vi "FTW-Example-SLASD-Core-Process.vi"() -> ()   [LabVIEW 2013, in "FTW-Example-SLASD-Core.lvclass"]
uses:
  FTW-Example-SLASD-Core.lvclass
  FTW-Example-SLASD-Core.lvclass/FTW-Example-SLASD-Core.ctl
  Actor/src/Instance/FTW-ActorInstance.lvclass/FTW-ActorInstance.ctl
  <vilib>/nisyscfg/Close (Hardware).vi
  <vilib>/nisyscfg/Close (System).vi
  <vilib>/nisyscfg/Find Hardware.vi
  Actor/src/JobSequencer/FTW-SEQ-Current.vi
  Actor/src/Instance/FTW-ActorInstance.lvclass
  Actor/src/Message/Request/FTW-Message-IncomingRequest.lvclass
  Actor/src/Ether/FTW-Ether.lvclass
  <vilib>/nisyscfg/nisyscfg.lvlib
  <resource>/objmgr/nisysapi.rc
panel:
  out "error out":errorcluster
  out "System Status":T1
  out "Elapsed Time":dbl format="%.6f sec"
  in  "Stop Button":bool
  # "avoid using Abort unless absolutely necessary"
  # "use this button to stop\nthe actor in RT dev mode\nsince user input events\ndo not work on RT"
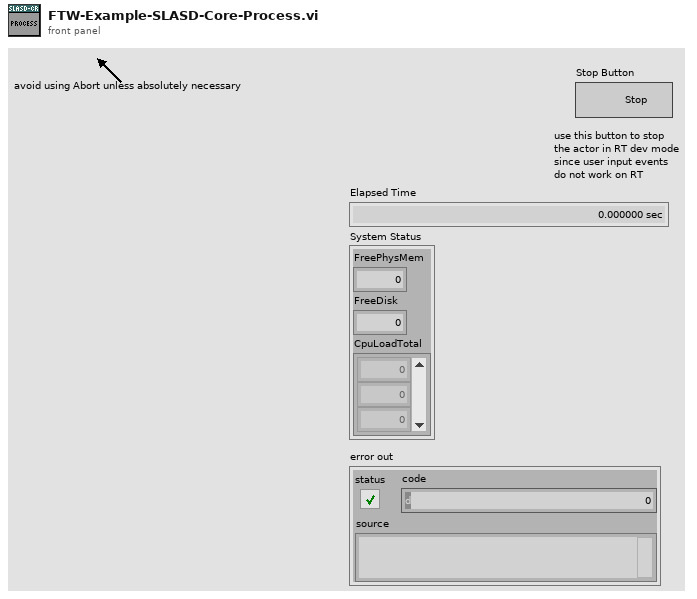
[diagram p1: front panel]
types:
  T1 = cluster{"FreePhysMem":dbl, "FreeDisk":dbl, "CpuLoadTotal":u32[]}
  T2 = cluster{"Incoming Requests":refnum<event-registration>, "Additional Registration Types":refnum<event-registration>}
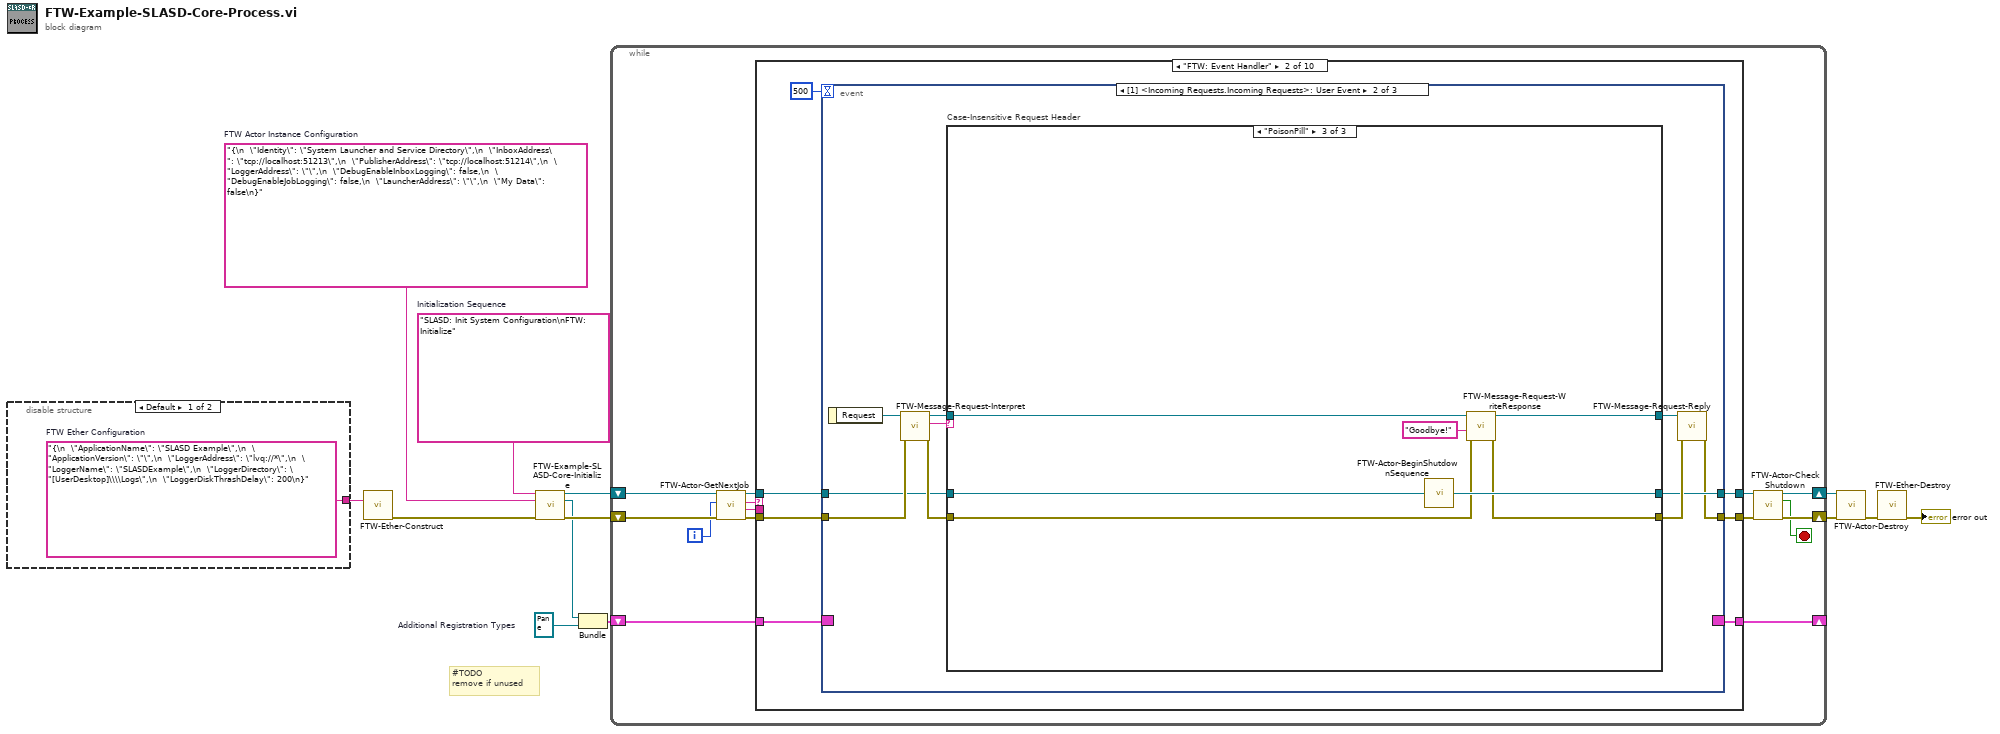
[diagram p0: block diagram]
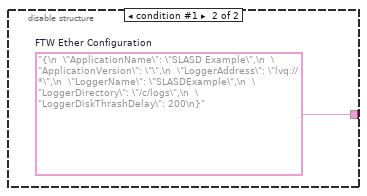
[diagram p2: hidden frame]
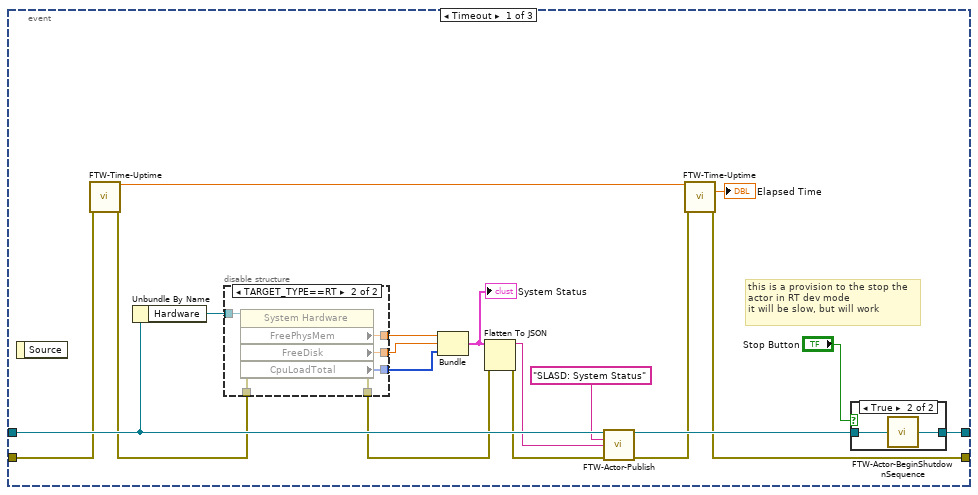
[diagram p4: hidden frame]
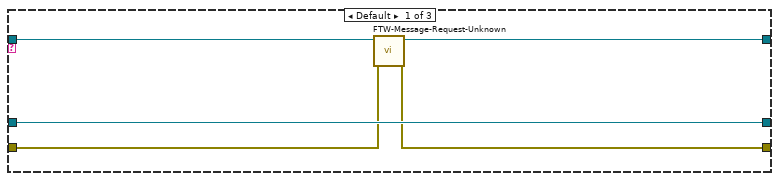
[diagram p7: hidden frame]
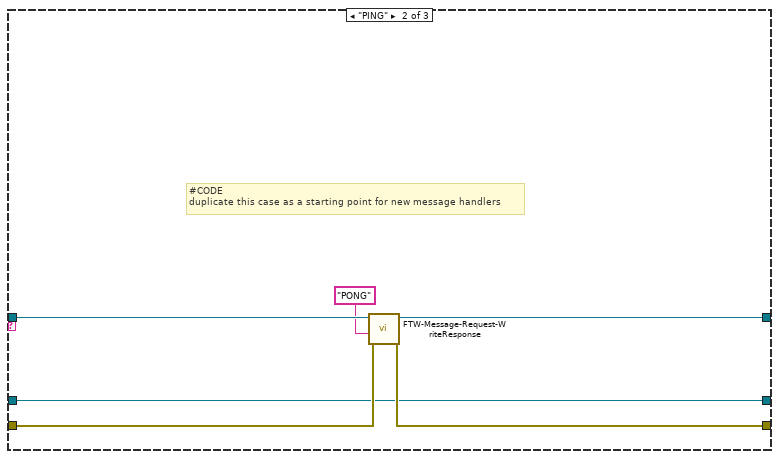
[diagram p8: hidden frame]
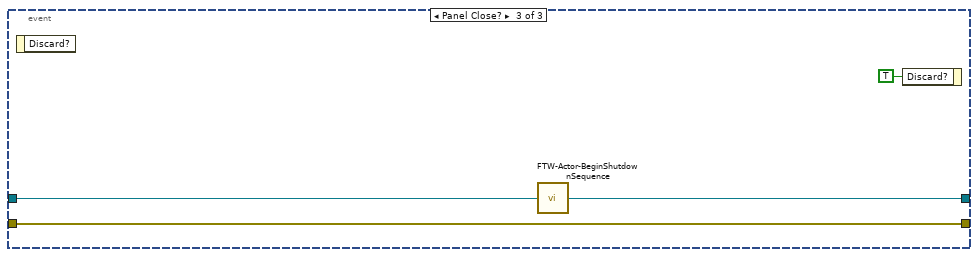
[diagram p9: hidden frame]
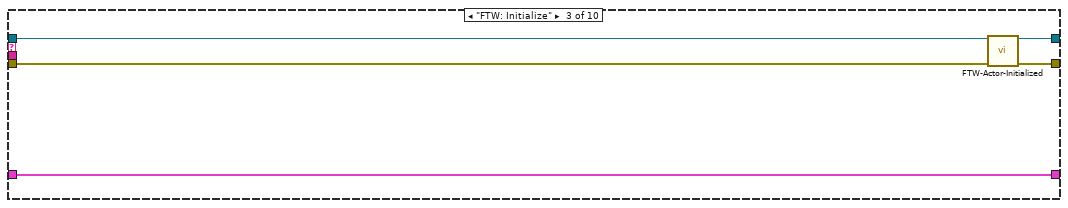
[diagram p10: hidden frame]
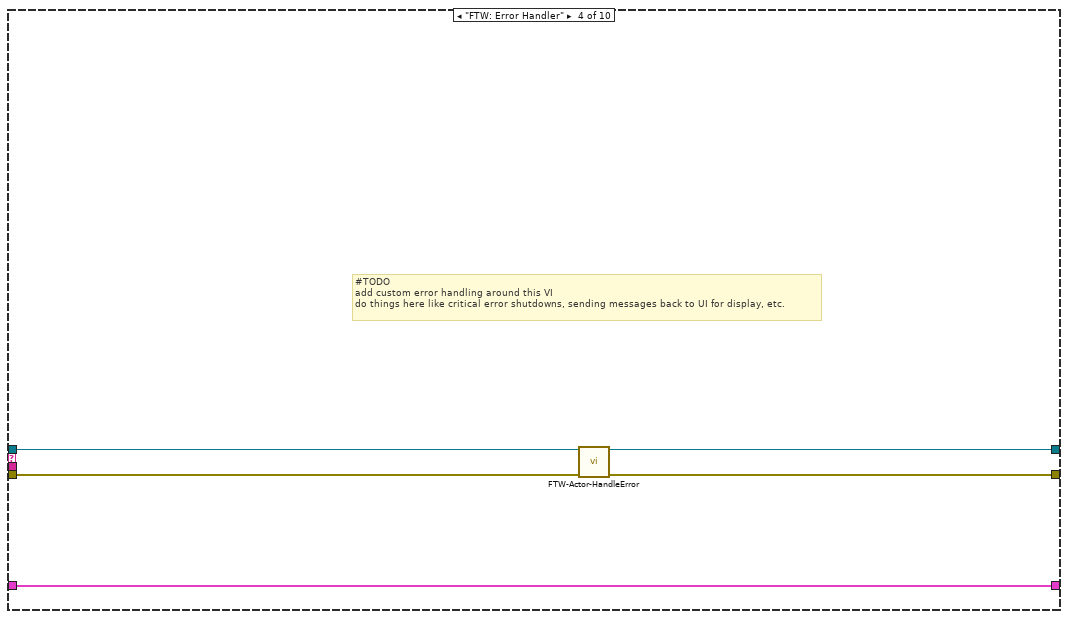
[diagram p11: hidden frame]
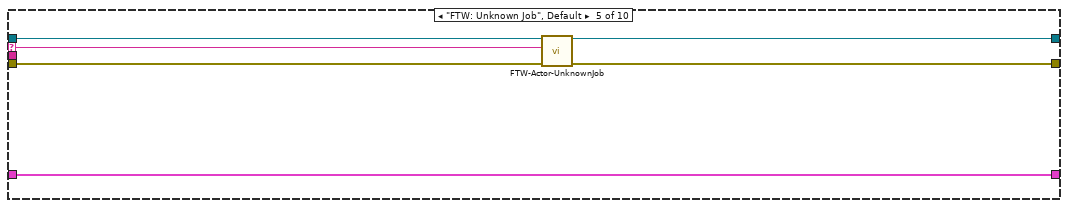
[diagram p12: hidden frame]
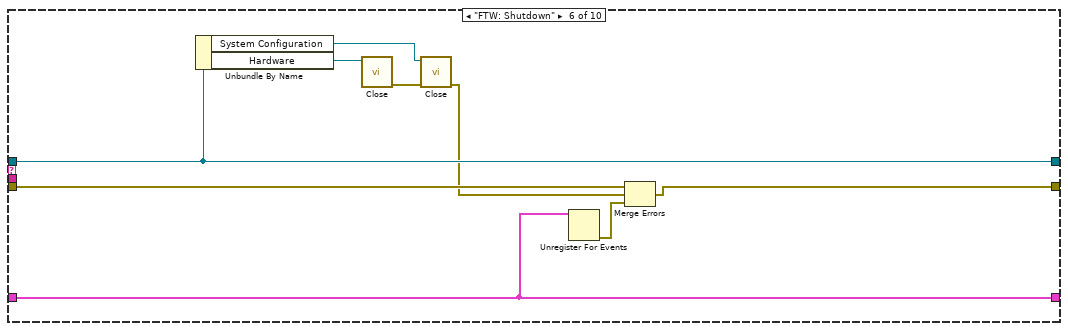
[diagram p13: hidden frame]
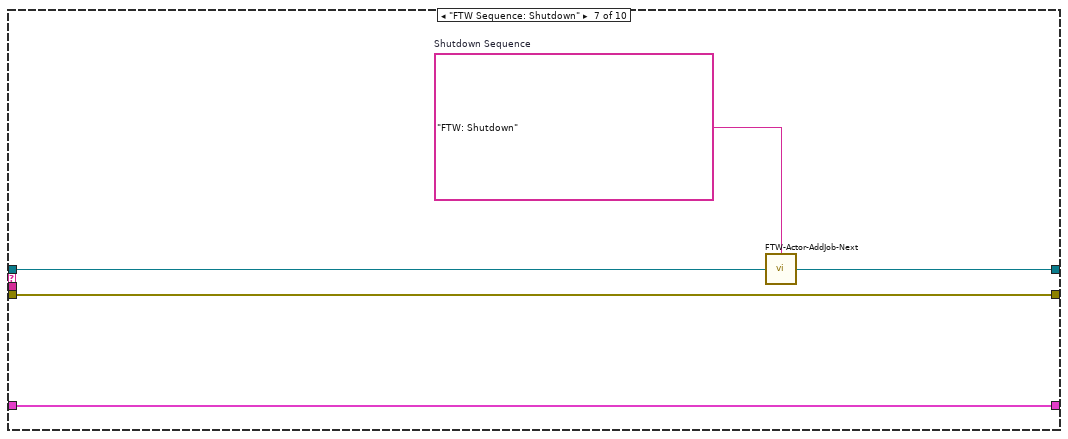
[diagram p14: hidden frame]
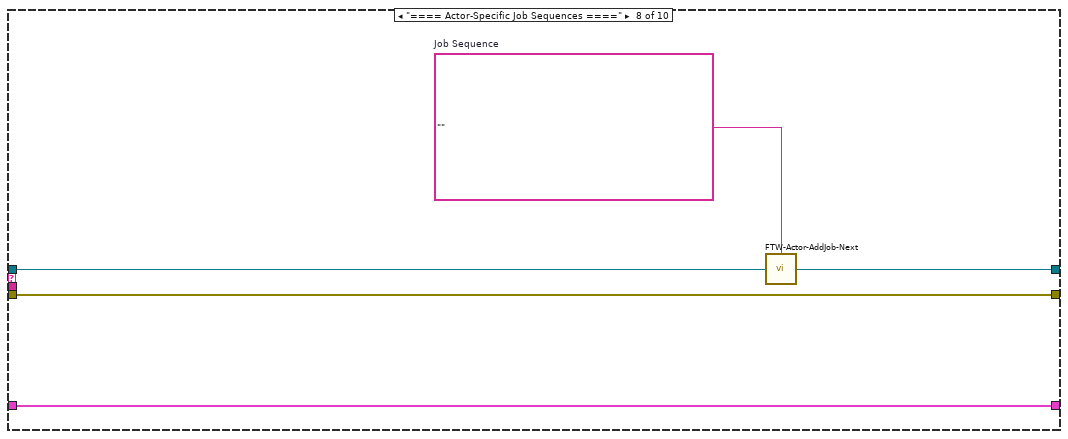
[diagram p15: hidden frame]
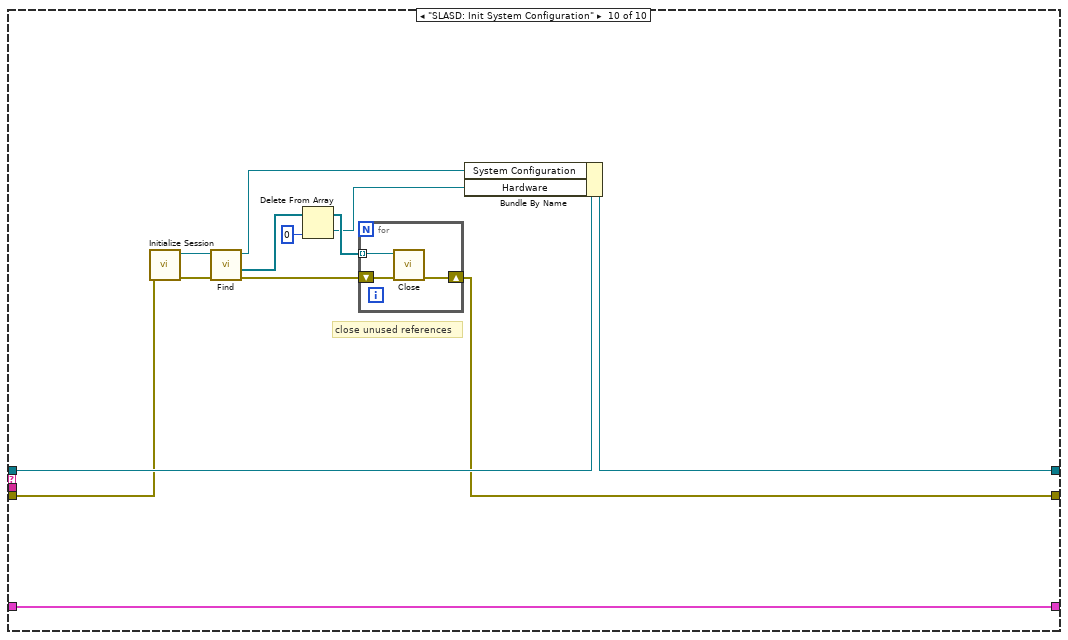
[diagram p17: hidden frame]
diagram:
  w5 = "{\n  \"Identity\": \"System Launcher and Service Directory\",\n  \"InboxAddress\": \"tcp://localhost:51213\",\n  \"PublisherAddress\": \"tcp://localhost:51214\",\n  \"LoggerAddress\": \"\",\n  \"DebugEnableInboxLogging\": false,\n  \"DebugEnableJobLogging\": false,\n  \"LauncherAddress\": \"\",\n  \"My Data\": false\n}"  # FTW Actor Instance Configuration
  w7 = refnum<event-registration> refnum  # Additional Registration Types
  w8 = "SLASD: Init System Configuration\nFTW: Initialize"  # Initialization Sequence
  # "#TODO\nremove if unused"
  n1 = disable-structure shown="Default" {
    disable-tunnel: [w14 w15] -> w2
    frame condition #0 (active) {
      w14 = "{\n  \"ApplicationName\": \"SLASD Example\",\n  \"ApplicationVersion\": \"\",\n  \"LoggerAddress\": \"lvq://*\",\n  \"LoggerName\": \"SLASDExample\",\n  \"LoggerDirectory\": \"[UserDesktop]\\\\Logs\",\n  \"LoggerDiskThrashDelay\": 200\n}"  # FTW Ether Configuration
    }
    frame condition #1 {
      w15 = "{\n  \"ApplicationName\": \"SLASD Example\",\n  \"ApplicationVersion\": \"\",\n  \"LoggerAddress\": \"lvq://*\",\n  \"LoggerName\": \"SLASDExample\",\n  \"LoggerDirectory\": \"/c/logs\",\n  \"LoggerDiskThrashDelay\": 200\n}"  # FTW Ether Configuration
    }
  }
  n2 = call "FTW-Ether-Construct.vi"("FTW Ether Configuration"=w2) -> ("error out"=w3:errorcluster)  [unwired: 14 in]
  n3 = call "FTW-Example-SLASD-Core-Initialize.vi"("Initialization Sequence"=w8, "FTW Actor Instance Configuration"=w5, "error in (no error)"=w3) -> ("Actor Template-Core out"=w13:refnum<class "FTW-Example-SLASD-Core.lvclass">, "Incoming Requests"=w4:refnum<event-registration>, "error out"=w9:errorcluster)  [unwired: 10 in]
  n4 = Bundle("Incoming Requests"=w4, "Additional Registration Types"=w7) -> (w6:T2)  [unwired: 1 in]
  n5 = while {
    shift-right: [w19] -> w11
    shift-left: w9 -> [w26]
    shift-right: [w16] -> _
    shift-left: w6 -> [w29]
    shift-right: [w21] -> w12
    shift-left: w13 -> [w28]
    i -> [w17]
    stop <- w18 stop-if-true
    n6 = call "FTW-Actor-GetNextJob.vi"("error in"=w26, "Jobs Performed"=w17, "FTW Actor Instance"=w28) -> ("error out"=w25:errorcluster, "Job Data"=w23:string, "Job Name"=w24:string, "FTW Actor Instance out"=w27:refnum<class "FTW-Example-SLASD-Core.lvclass">)  [unwired: 5 in]
    n7 = case shown="\"FTW: Event Handler\"" w24 {
      selector: w24 -> [_ _ _ _ w111 _ _ _ _ _]
      tunnel: [w31 w39 w101 w106 w114 w124 w129 w134 w138 w142] -> w20
      tunnel: w25 -> [w31 w38 w104 w108 w115 w125 w129 w134 w138 w143]
      tunnel: w29 -> [w32 w34 w105 w110 w116 w122 w130 w135 w137 w151]
      tunnel: [w32 w37 w105 w110 w116 w122 w130 w135 w137 w151] -> w16
      tunnel: w23 -> [_ _ _ _ _ _ _ _ _ _]
      tunnel: [w30 w36 w102 w107 w112 w121 w127 w132 w136 w141] -> w22
      tunnel: w27 -> [w30 w35 w103 w109 w113 w121 w128 w133 w136 w150]
      frame "==== Featherweight Framework Jobs ====" {
      }
      frame "FTW: Event Handler" {
        n8 = event shown="[1] <Incoming Requests.Incoming Requests>: User Event" {
          selector: w34 -> [_ _ _]
          dyn-events: [_ _ _] -> w37
          timeout: 500 -> [_ _ _]
          tunnel: [w42 w71 w99] -> w39
          tunnel: w38 -> [w56 w70 w99]
          tunnel: [w45 w72 w97] -> w36
          tunnel: w35 -> [w58 w69 w98]
          event Timeout {
            # "this is a provision to the stop the\nactor in RT dev mode\nit will be slow, but will work"
            n9 = event-data() -> ()  [unwired: 1 in, 1 out]
            n10 = call "FTW-Time-Uptime.vi"("error in"=w56) -> ("Current Uptime"=w41:dbl, "error out"=w43:errorcluster)  [unwired: 12 in, 1 out]
            n11 = Unbundle By Name(w58) -> ("Hardware"=w57:refnum<k20>)
            n12 = disable-structure shown="TARGET_TYPE==RT" {
              disable-tunnel: w43 -> [w62 w68]
              disable-tunnel: [_ w67] -> w50
              disable-tunnel: w57 -> [_ w66]
              disable-tunnel: [_ w65] -> w51
              disable-tunnel: [_ w64] -> w52
              disable-tunnel: [w62 w63] -> w49
              frame condition #0 (active) {
              }
              frame condition #1 {
                n13 = property class="System Hardware"(reference=w66, error in=w68) -> (error out=w63:errorcluster, "FreePhysMem"=w64:dbl, "FreeDisk"=w65:dbl, "CpuLoadTotal"=w67:u32[])  [unwired: 1 out]
              }
            }
            n14 = Bundle("FreePhysMem"=w52, "FreeDisk"=w51, "CpuLoadTotal"=w50) -> (w47:T1)  [unwired: 1 in]
            "System Status" <- w47
            n15 = Flatten To JSON(anything=w47, error in (no error)=w49) -> (JSON string=w46:string, 11:w48:errorcluster)  [unwired: 1 in]
            n16 = call "FTW-Actor-Publish.vi"("FTW-ActorInstance In"=w58, "Message Header"="SLASD: System Status", "Message Body"=w46, "error in (no error)"=w48) -> ("FTW-ActorInstance Out"=w55:refnum<class "FTW-Example-SLASD-Core.lvclass">, "error out"=w54:errorcluster)  [unwired: 10 in]
            n17 = call "FTW-Time-Uptime.vi"("Previous Uptime"=w41, "error in"=w54) -> ("Elapsed Time"=→"Elapsed Time":dbl, "error out"=w42:errorcluster)  [unwired: 11 in, 1 out]
            n18 = case shown="True" "Stop Button" {
              tunnel: w55 -> [w59 w61]
              tunnel: [w59 w60] -> w45
              frame False {
              }
              frame True {
                n19 = call "FTW-Actor-BeginShutdownSequence.vi"("FTW Actor Instance"=w61) -> ("FTW Actor Instance out"=w60:refnum<class "FTW-Example-SLASD-Core.lvclass">)  [unwired: 3 in]
              }
            }
          }
          event User Event {
            n20 = event-data() -> ("Request"=w73:refnum<class "FTW-Message-IncomingRequest.lvclass">)  [unwired: 1 in]
            n21 = call "FTW-Message-Request-Interpret.vi"("error in"=w70, "FTW Incoming Request"=w73) -> ("error out"=w78:errorcluster, "Request Header"=w76:string, "FTW Incoming Request out"=w75:refnum<class "FTW-Message-IncomingRequest.lvclass">)  [unwired: 7 in]
            n22 = case "Case-Insensitive Request Header" shown="\"PoisonPill\"" w76 {
              tunnel: [w81 w87 w93] -> w77
              tunnel: w78 -> [w82 w88 w95]
              tunnel: [w83 w86 w96] -> w72
              tunnel: w69 -> [w83 w86 w94]
              tunnel: w75 -> [w80 w89 w92]
              tunnel: [w79 w85 w91] -> w74
              frame Default {
                n23 = call "FTW-Message-Request-Unknown.vi"("error in"=w82, "FTW Incoming Request"=w80) -> ("error out"=w81:errorcluster, "FTW Incoming Request Out"=w79:refnum<class "FTW-Message-IncomingRequest.lvclass">)  [unwired: 8 in]
              }
              frame "PING" {
                # "#CODE\nduplicate this case as a starting point for new message handlers"
                n24 = call "FTW-Message-Request-WriteResponse.vi"("error in"=w88, "Response Body"="PONG" ("Response Header"), "FTW Incoming Request"=w89) -> ("error out"=w87:errorcluster, "FTW Incoming Request out"=w85:refnum<class "FTW-Message-IncomingRequest.lvclass">)  [unwired: 7 in]
              }
              frame "PoisonPill" {
                n25 = call "FTW-Actor-BeginShutdownSequence.vi"("FTW Actor Instance"=w94) -> ("FTW Actor Instance out"=w96:refnum<class "FTW-Example-SLASD-Core.lvclass">)  [unwired: 3 in]
                n26 = call "FTW-Message-Request-WriteResponse.vi"("error in"=w95, "Response Body"="Goodbye!", "FTW Incoming Request"=w92) -> ("error out"=w93:errorcluster, "FTW Incoming Request out"=w91:refnum<class "FTW-Message-IncomingRequest.lvclass">)  [unwired: 7 in]
              }
            }
            n27 = call "FTW-Message-Request-Reply.vi"("error in"=w77, "FTW Incoming Request"=w74) -> ("error out"=w71:errorcluster)  [unwired: 8 in, 1 out]
          }
          event Panel Close? {
            n28 = event-data() -> ()  [unwired: 1 in, 1 out]
            n29 = call "FTW-Actor-BeginShutdownSequence.vi"("FTW Actor Instance"=w98) -> ("FTW Actor Instance out"=w97:refnum<class "FTW-Example-SLASD-Core.lvclass">)  [unwired: 3 in]
            n30 = event-data("Discard?"=TRUE) -> ()  [unwired: 1 in, 1 out]
          }
        }
      }
      frame "FTW: Initialize" {
        n31 = call-dynamic "FTW-Actor-Initialized.vi"("FTW Actor Instance"=w103, "error in"=w104) -> ("FTW Actor Instance out"=w102:refnum<class "FTW-Example-SLASD-Core.lvclass">, "error out"=w101:errorcluster)  [unwired: 12 in]
      }
      frame "FTW: Error Handler" {
        # "#TODO\nadd custom error handling around this VI\ndo things here like critical error shutdowns, sending messages back to UI for display, etc."
        n32 = call-dynamic "FTW-Actor-HandleError.vi"("FTW Actor Instance"=w109, "error in"=w108) -> ("FTW Actor Instance out"=w107:refnum<class "FTW-Example-SLASD-Core.lvclass">, "error out"=w106:errorcluster)  [unwired: 11 in, 1 out]
      }
      frame "FTW: Unknown Job", Default {
        n33 = call-dynamic "FTW-Actor-UnknownJob.vi"("FTW Actor Instance"=w113, "Unknown Job"=w111, "error in"=w115) -> ("FTW Actor Instance out"=w112:refnum<class "FTW-Example-SLASD-Core.lvclass">, "error out"=w114:errorcluster)  [unwired: 11 in]
      }
      frame "FTW: Shutdown" {
        n34 = Unbundle By Name(w121) -> ("System Configuration"=w118:refnum<k21>, "Hardware"=w120:refnum<k20>)
        n35 = call-poly <vilib>:"Close.vi"("resource in"=w120) -> ("error out"=w119:errorcluster)  [unwired: 10 in]
        n36 = call-poly <vilib>:"Close.vi"("error in (no error)"=w119, "session in"=w118) -> ("error out"=w117:errorcluster)  [unwired: 9 in]
        n37 = Unregister For Events(event registration refnum=w122) -> (error out=w123:errorcluster)  [unwired: 1 in]
        n38 = Merge Errors(w125, w117, w123) -> (w124:errorcluster)
      }
      frame "FTW Sequence: Shutdown" {
        w126 = "FTW: Shutdown"  # Shutdown Sequence
        n39 = call "FTW-Actor-AddJob-Next.vi"("Add Next in Job Queue"=w126, "FTW Actor Instance"=w128) -> ("FTW Actor Instance out"=w127:refnum<class "FTW-Example-SLASD-Core.lvclass">)  [unwired: 2 in]
      }
      frame "==== Actor-Specific Job Sequences ====" {
        w131 = ""  # Job Sequence
        n40 = call "FTW-Actor-AddJob-Next.vi"("Add Next in Job Queue"=w131, "FTW Actor Instance"=w133) -> ("FTW Actor Instance out"=w132:refnum<class "FTW-Example-SLASD-Core.lvclass">)  [unwired: 2 in]
      }
      frame "==== Actor-Specific Jobs ====" {
      }
      frame "SLASD: Init System Configuration" {
        # "close unused references"
        n41 = call <vilib>:"Initialize Session.vi"("error in (no error)"=w143) -> ("error out"=w149:errorcluster, "session out"=w148:refnum<k21>)  [unwired: 9 in]
        n42 = call-poly <vilib>:"Find.vi"("error in (no error)"=w149, "session in"=w148) -> ("error out"=w145:errorcluster, "resources out"=w147:refnum<k20>[], "session out"=w140:refnum<k21>)  [unwired: 6 in, 1 out]
        n43 = Delete From Array(array=w147, index=0) -> (deleted portion=w139:refnum<k20>, array with subset deleted=w144:refnum<k20>[])  [unwired: 1 in]
        n44 = for {
          tunnel: w144 -> [w154] mode=indexing
          shift-right: [w152] -> w142
          shift-left: w145 -> [w153]
          n45 = call-poly <vilib>:"Close.vi"("error in (no error)"=w153, "resource in"=w154) -> ("error out"=w152:errorcluster)  [unwired: 9 in]
        }
        n46 = Bundle By Name(cluster=w150, "System Configuration"=w140, "Hardware"=w139) -> (w141:refnum<class "FTW-Example-SLASD-Core.lvclass">)
      }
    }
    n47 = call "FTW-Actor-CheckShutdown.vi"("FTW Actor Instance"=w22, "error in"=w20) -> ("FTW Actor Instance out"=w21:refnum<class "FTW-Example-SLASD-Core.lvclass">, "Shutdown?"=w18:bool, "error out"=w19:errorcluster)  [unwired: 11 in]
  }
  n48 = call-dynamic "FTW-Actor-Destroy.vi"("FTW Actor Instance"=w12, "error in"=w11) -> ("error out"=w10:errorcluster)  [unwired: 13 in]
  n49 = call "FTW-Ether-Destroy.vi"("error in"=w10) -> ("error out"=→"error out":errorcluster)  [unwired: 14 in]
